vi "panel1.vi"(8 "error in (no error)":errorcluster) -> (0 "error out":errorcluster)   [LabVIEW 2017]
uses:
  bb6a7318-aad0-43dc-afe4-77ceae751020.vi
  bc86f585-7601-4354-b9cf-83381ec6f4b2.vi
  2c6c05eb-32f5-4c4c-892e-8fac7bb5f8bf.vi
  TagDB/_Support/DataAccess/data-Write.vi
  TagDB/_Support/DataAccess/_NameCacher.vi
  TagDB/_Support/DataAccess/_datatypeChecker.vi
  TagDB/_Support/DataAccess/TagDB Ref to DVR.vi
  <vilib>/Utility/Data Type/Get Type Information.vi
  <vilib>/Utility/error.llb/Trim Whitespace.vi
  TagDB/_Support/Error/_[error50000]Invalid DB REF.vi
  TagDB/_Support/URL/TRIM-BOTH-SPACE.vi
  TagDB/_Support/Error/_[error50002]Invalid DataType.vi
  TagDB/TagDB.lvlib
panel:
  in  "abcdef":T1={"number"=0, "boolean"=TRUE, "abcdef"={"number"=0, "boolean"=TRUE}}
  in  "value":string="test send message"
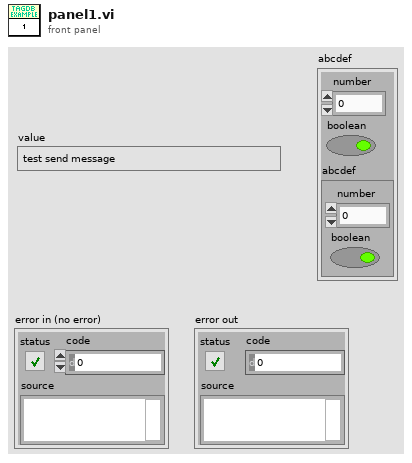
[diagram p1: front panel]
types:
  T1 = cluster{"number":i32, "boolean":bool, "abcdef":cluster{"number":i32, "boolean":bool}}
  T2 = typedef "TagDB.lvlib/TagDB.ctl" = refnum<k1>
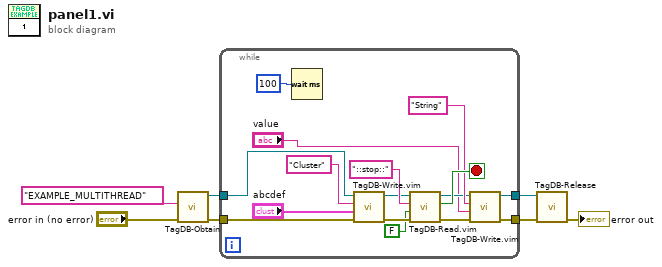
[diagram p0: block diagram]
diagram:
  n1 = call "TagDB-Obtain.vi"("error in (no error)"="error in (no error)", "name (unnamed)"="EXAMPLE_MULTITHREAD") -> ("error out"=w5:errorcluster, "TagDB"=w4:T2)  [unwired: 3 in, 1 out]
  n2 = while {
    tunnel: w4 -> [w12]
    tunnel: w5 -> [w10]
    tunnel: [w16] -> w7
    tunnel: [w19] -> w1
    stop <- w21 stop-if-true
    n3 = Wait (ms)(milliseconds to wait=u32 100) -> ()  [unwired: 1 out]
    n4 = call "TagDB-Write.vim"("error in (no error)"=w10, "Value"="abcdef", "name"="Cluster", "TagDB"=w12) -> ("error out"=w9:errorcluster, "TagDB(dup)"=w11:T2)  [unwired: 5 in, 1 out]
    n5 = call "TagDB-Read.vim"("error in (no error)"=w9, "Type(empty to read as variant)"=FALSE, "name"="::stop::", "TagDB"=w11) -> ("error out"=w18:errorcluster, "Value"=w21:bool, "TagDB(dup)"=w17:T2)  [unwired: 2 in, 3 out]
    n6 = call "TagDB-Write.vim"("error in (no error)"=w18, "Value"="value", "name"="String", "TagDB"=w17) -> ("error out"=w16:errorcluster, "TagDB(dup)"=w19:T2)  [unwired: 5 in, 1 out]
  }
  n7 = call "TagDB-Release.vi"("error in (no error)"=w7, "TagDB"=w1) -> ("error out"=→"error out":errorcluster)  [unwired: 9 in]
